vi "Proverka(0).vi"(11 "all rows":string[][](array[string])=[["", "50000", "100000", "200000"], ["100", "0", "0", "0"], ["75.3", "-11.3", "-21.7", "-46.55"], ["55.3", "-19.9", "-30.2", "-69.65"], ["35.3", "-30", "-47.2", "-109.2"], ["", "", "", ""], ["", "", "", ""], ["", "", "", ""]]) -> (1 "ArrayChastot":dbl[][](array[numeric]), 2 "All GLUBIN":dbl[](array[numeric]), 3 "x >= 0?":bool)   [LabVIEW 2017]
panel:
  out "Chastota":dbl[](array[numeric])
  out "ZnachChastot":dbl[](array[numeric])
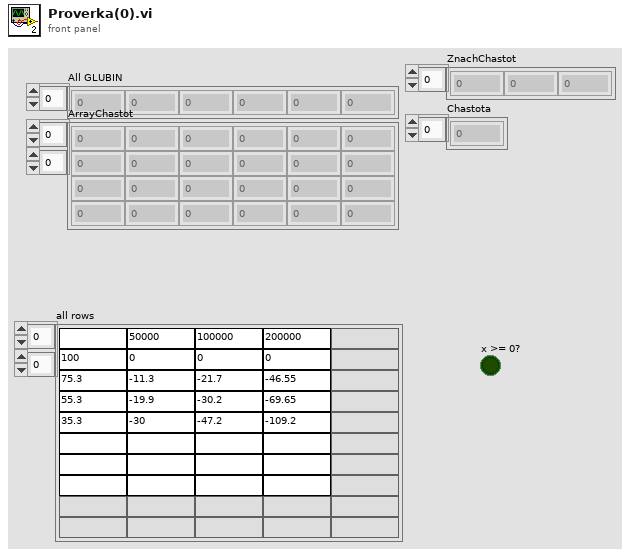
[diagram p1: front panel]
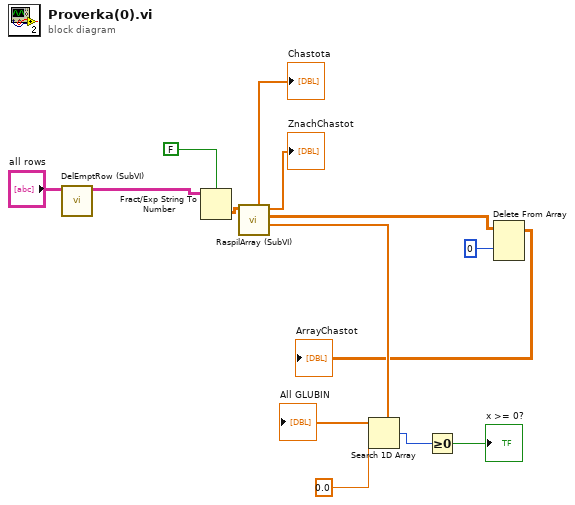
[diagram p0: block diagram]
diagram:
  n1 = call "DelEmptRow (SubVI).vi"("all rows in"="all rows") -> ("all rows out"=w9:string[][])  [unwired: 10 in]
  n2 = Fract/Exp String To Number(use system decimal point (T)=FALSE, string=w9) -> (number=w12:dbl[][])  [unwired: 2 in, 1 out]
  n3 = call "RaspilArray (SubVI).vi"("Array 3"=w12) -> ("All GLUBIN"=w7:dbl[], "Array 2"=w3:dbl[][], "ZnachChastot"=→"ZnachChastot":dbl[], "Chastota"=→"Chastota":dbl[])  [unwired: 6 in, 1 out]
  "All GLUBIN" <- w7
  n4 = Search 1D Array(1D array=w7, element=0.0) -> (index of element=w5:i32)  [unwired: 1 in]
  n5 = Greater Or Equal To 0?(x=w5) -> (x >= 0?=→"x >= 0?":bool)
  n6 = Delete From Array(array=w3, index (row)=0) -> (array with subset deleted=→"ArrayChastot":dbl[][])  [unwired: 2 in, 1 out]
